vi "BuildMDF.vi"() -> ()   [LabVIEW 2010]
panel:
  out "Draw??":bool
  in  "MDFile":T1
  out "initialized MDF":T2(array[cluster])
  in  "sset/reset MDF":bool
  out "MDF_Original":T2(array[cluster])
  in  "2D Picture":picture
  out "NewMissionDefMap":picture
  in  "Build MDF":bool
  in  "Select Pen Attributes":T3={"Width"=1, "Style"=enum."Solid"}
  in  "Select Your Behavior":T4(ring)
  out "No. of Waypoints":i32
  in  "Path Leg Depth":dbl
  in  "Path Leg Speed":dbl
  out "MissionDefFile":picture
  in  "Pen Color":u32(colorbox)=15671808
  out "Way Point Index":i32
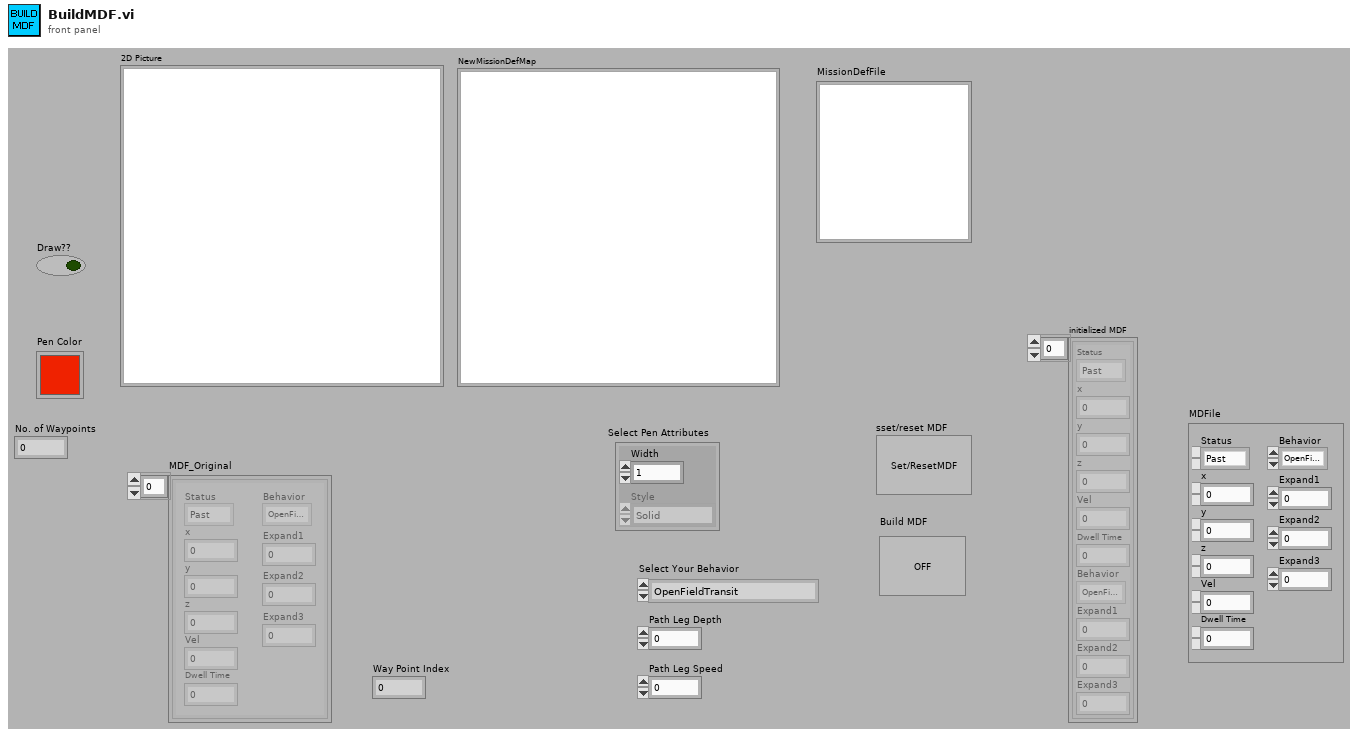
[diagram p1: front panel]
types:
  T1 = cluster{"Status":enum16{"Past", "Current", "Future"}, "x":dbl, "y":dbl, "z":dbl, "Vel":dbl, "Dwell Time":dbl, "Behavior":enum16{"OpenFieldTransit", "WallFollow", "LaneFollow", "ManualMode"}, "Expand1":dbl, "Expand2":dbl, "Expand3":dbl}
  T2 = cluster{"Status":enum16{"Past", "Current", "Future"}, "x":dbl, "y":dbl, "z":dbl, "Vel":dbl, "Dwell Time":dbl, "Behavior":enum16{"OpenFieldTransit", "WallFollow", "LaneFollow", "ManualMode"}, "Expand1":dbl, "Expand2":dbl, "Expand3":dbl}[]
  T3 = cluster{"Width":u16, "Style":enum32{"Solid", "Dash", "Dot", "DashDot", "DashDotDot"}}
  T4 = enum16{"OpenFieldTransit", "WallFollow", "LaneFollow", "ManualMode"}
  T5 = cluster{"Status":enum16{"Past", "Current", "Future"}, "x":dbl, "y":dbl, "z":dbl, "Vel":dbl, "Dwell Time":dbl, "Behavior":enum16{"OpenWaterTransit", "WallFollow", "LaneFollow", "Stop"}, "Expand1":dbl, "Expand2":dbl, "Expand3":dbl}[]
  T6 = enum32{"Solid", "Dash", "Dot", "DashDot", "DashDotDot"}
  T7 = typedef "LVMouseTypeDef.ctl" = cluster{"Mouse Position":cluster{"X":i32, "Y":i32}, "Mouse Modifiers":cluster{"Button Down":bool, "Shift Mod":bool, "Menu Mod":bool, "Option Mod":bool}}
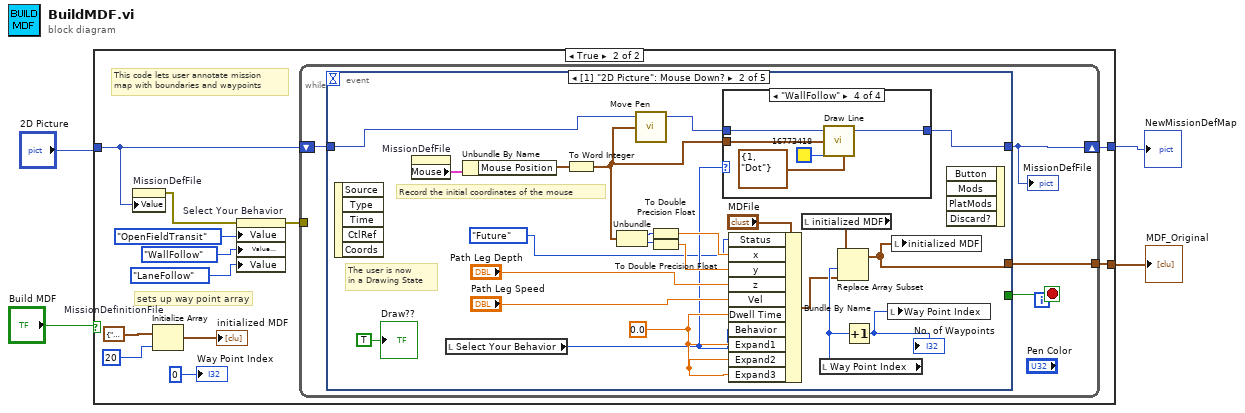
[diagram p0: block diagram]
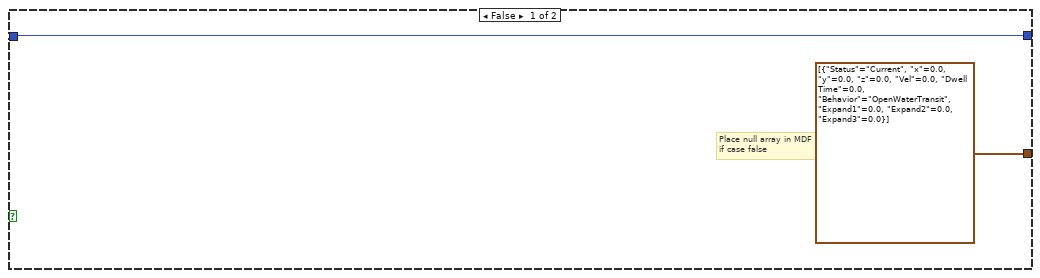
[diagram p2: hidden frame]
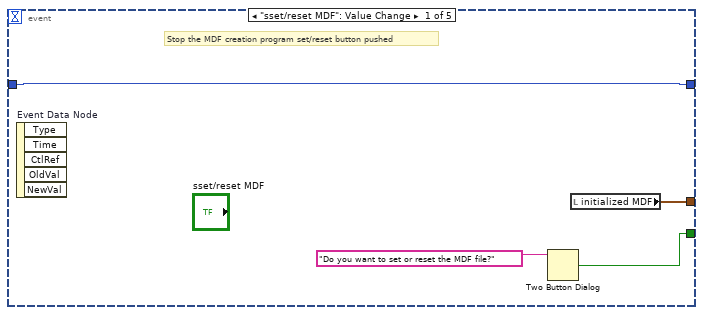
[diagram p3: hidden frame]
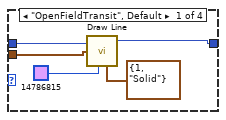
[diagram p4: hidden frame]
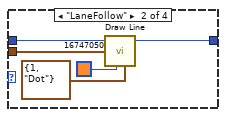
[diagram p5: hidden frame]
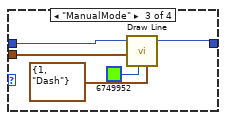
[diagram p6: hidden frame]
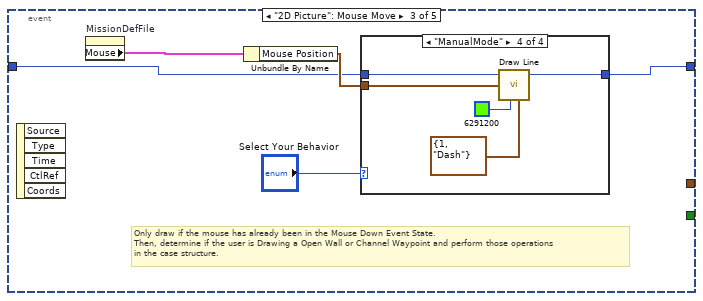
[diagram p7: hidden frame]
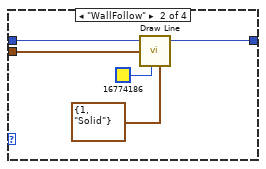
[diagram p9: hidden frame]
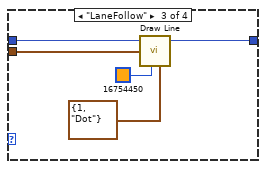
[diagram p10: hidden frame]
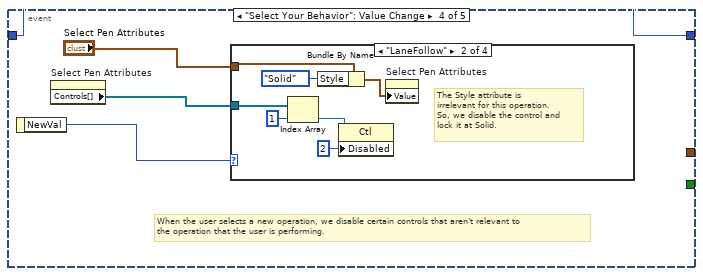
[diagram p11: hidden frame]
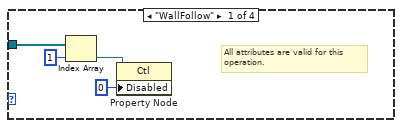
[diagram p12: hidden frame]
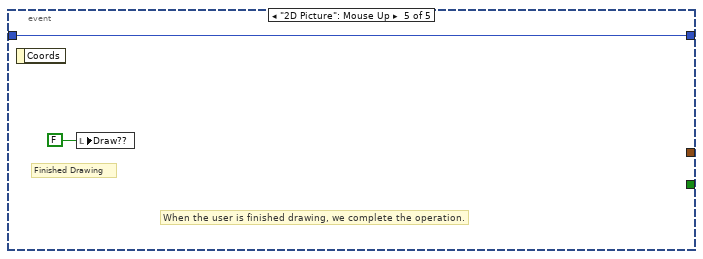
[diagram p15: hidden frame]
diagram:
  n1 = case shown="True" "Build MDF" {
    tunnel: "2D Picture" -> [w6 w16]
    tunnel: [w6 w13] -> w3
    tunnel: [T5 [{"Status"=enum."Current", "x"=0.0, "y"=0.0, "z"=0.0, "Vel"=0.0, "Dwell Time"=0.0, "Behavior"=enum."OpenWaterTransit", "Expand1"=0.0, "Expand2"=0.0, "Expand3"=0.0}] ("MDF_Original") w10] -> w1
    frame False {
      # "Place null array in MDF\nif case false"
    }
    frame True {
      w12 = T1 {"Status"=enum."Current", "x"=0.0, "y"=0.0, "z"=0.0, "Vel"=0.0, "Dwell Time"=0.0, "Behavior"=enum."OpenFieldTransit", "Expand1"=0.0, "Expand2"=0.0, "Expand3"=0.0}  # MissionDefinitionFile
      # "sets up way point array"
      # "This code lets user annotate mission\nmap with boundaries and waypoints"
      n2 = property on="MissionDefFile" class="Pict"("Value"=w16) -> (error out=w17:errorcluster)  [unwired: 2 in, 1 out]
      n3 = Initialize Array ("Initialize WaypointArray")(w12, 20 ("dimension size")) -> (→"initialized MDF":T2)
      n4 = property on="Select Your Behavior" class="Enum (strict)"(error in=w17, "Value"=T4."OpenFieldTransit" ("Select Your Behavior"), "Value (Signaling)"=T4."WallFollow", "Value"=T4."LaneFollow" ("Select Your Behavior")) -> (error out=w18:errorcluster)  [unwired: 1 in, 1 out]
      n5 = while {
        shift-right: [w19] -> w13
        shift-left: w16 -> [w21]
        tunnel: w18 -> [_]
        tunnel: [w20] -> w10
        stop <- w22 stop-if-true
        n6 = event shown="[1] \"2D Picture\": Mouse Down?" {
          selector: _ -> [_ _ _ _ _]
          dyn-events: _ -> [_ _ _ _ _]
          timeout: _ -> [_ _ _ _ _]
          tunnel: [w26 w45 w69 w92 _] -> w19
          tunnel: w21 -> [w26 w43 w70 w92 w106]
          tunnel: [w24 _ _ _ _] -> w22
          tunnel: [w23 w42 _ _ _] -> w20
          tunnel: [_ _ _ _ w106] -> _
          event "sset/reset MDF": Value Change {
            # "Stop the MDF creation program set/reset button pushed"
            n7 = event-data "Event Data Node"() -> ()  [unwired: 1 in, 5 out]
            n8 = Two Button Dialog(message="Do you want to set or reset the MDF file?") -> (T button?=w24:bool)  [unwired: 2 in]
            n9 = local read "initialized MDF"() -> (w23:T2)
          }
          event "2D Picture": Mouse Down? {
            w31 = 0.0 ("Dwell Time")
            # "Record the initial coordinates of the mouse"
            # "The user is now\nin a Drawing State"
            n10 = event-data() -> ()  [unwired: 1 in, 5 out]
            n11 = property on="MissionDefFile" class="Pict"() -> ("Mouse"=w48:T7)  [unwired: 2 in, 2 out]
            n12 = local read "Select Your Behavior"() -> (w30:T4)
            n13 = Unbundle By Name(w48) -> ("Mouse Position"=w44:cluster{"X":i32, "Y":i32})
            n14 = To Word Integer(number=w44) -> (16bit integer=w29:cluster{"X":i16, "Y":i16})
            n15 = Unbundle(w29) -> ("X"=w37:i16, "Y"=w36:i16)
            n16 = call <vilib>:"Move Pen.vi"("new position"=w29, "picture"=w43) -> ("new picture"=w47:picture)  [unwired: 3 in]
            n17 = To Double Precision Float(number=w37) -> (double precision float=w35:dbl)
            n18 = To Double Precision Float(number=w36) -> (double precision float=w34:dbl)
            n19 = case shown="\"WallFollow\"" w30 {
              tunnel: w47 -> [w53 w58 w61 w66]
              tunnel: [w52 w54 w59 w64] -> w45
              tunnel: w29 -> [w51 w57 w60 w65]
              frame "OpenFieldTransit", Default {
                n20 = call <vilib>:"Draw Line.vi"("picture"=w53, "end point"=w51, "color(black)"=u32 14786815, "pen"=T3 {"Width"=1, "Style"=enum."Solid"}) -> ("new picture"=w52:picture)  [unwired: 5 in]
              }
              frame "LaneFollow" {
                n21 = call <vilib>:"Draw Line.vi"("picture"=w58, "end point"=w57, "color(black)"=u32 16747050, "pen"=T3 {"Width"=1, "Style"=enum."Dot"}) -> ("new picture"=w54:picture)  [unwired: 5 in]
              }
              frame "ManualMode" {
                n22 = call <vilib>:"Draw Line.vi"("picture"=w61, "end point"=w60, "color(black)"=u32 6749952, "pen"=T3 {"Width"=1, "Style"=enum."Dash"}) -> ("new picture"=w59:picture)  [unwired: 5 in]
              }
              frame "WallFollow" {
                n23 = call <vilib>:"Draw Line.vi"("picture"=w66, "end point"=w65, "color(black)"=u32 16773418, "pen"=T3 {"Width"=1, "Style"=enum."Dot"}) -> ("new picture"=w64:picture)  [unwired: 5 in]
              }
            }
            n24 = Bundle By Name(cluster="MDFile", "Status"=enum16{"Past", "Current", "Future"}."Future", "x"=w35, "y"=w34, "z"="Path Leg Depth", "Vel"="Path Leg Speed", "Dwell Time"=w31, "Behavior"=w30, "Expand1"=w31, "Expand2"=w31, "Expand3"=w31) -> (w38:T1)
            n25 = local read "initialized MDF"() -> (w40:T2)
            n26 = local read "Way Point Index"() -> (w41:i32)
            n27 = Replace Array Subset(array=w40, new element=w38, index=w41) -> (w42:T2)
            n28 = Increment(x=w41) -> (x+1=w46:i32)
            "No. of Waypoints" <- w46
            n29 = local write "Way Point Index"(w46) -> ()
            n30 = local write "initialized MDF"(w42) -> ()
            n31 = event-data() -> ()  [unwired: 5 in, 1 out]
            "Draw??" <- TRUE ("Draw??")
          }
          event "2D Picture": Mouse Move {
            # "Only draw if the mouse has already been in the Mouse Down Event State.\nThen, determine if the user is Drawing a Open Wall or Channel Waypoint and perform those operations\nin the case structure."
            n32 = event-data() -> ()  [unwired: 1 in, 5 out]
            n33 = property on="MissionDefFile" class="Pict"() -> ("Mouse"=w73:T7)  [unwired: 2 in, 2 out]
            n34 = Unbundle By Name(w73) -> ("Mouse Position"=w71:cluster{"X":i32, "Y":i32})
            n35 = case shown="\"ManualMode\"" "Select Your Behavior" {
              tunnel: w71 -> [_ w78 w83 w86]
              tunnel: [w74 w79 w84 w85] -> w69
              tunnel: w70 -> [w74 w77 w80 w87]
              frame "OpenFieldTransit", Default {
              }
              frame "WallFollow" {
                n36 = call <vilib>:"Draw Line.vi"("picture"=w77, "end point"=w78, "color(black)"=u32 16774186, "pen"=T3 {"Width"=1, "Style"=enum."Solid"}) -> ("new picture"=w79:picture)  [unwired: 5 in]
              }
              frame "LaneFollow" {
                n37 = call <vilib>:"Draw Line.vi"("picture"=w80, "end point"=w83, "color(black)"=u32 16754450, "pen"=T3 {"Width"=1, "Style"=enum."Dot"}) -> ("new picture"=w84:picture)  [unwired: 5 in]
              }
              frame "ManualMode" {
                n38 = call <vilib>:"Draw Line.vi"("picture"=w87, "end point"=w86, "color(black)"=u32 6291200, "pen"=T3 {"Width"=1, "Style"=enum."Dash"}) -> ("new picture"=w85:picture)  [unwired: 5 in]
              }
            }
          }
          event "Select Your Behavior": Value Change {
            # "When the user selects a new operation, we disable certain controls that aren't relevant to\nthe operation that the user is performing."
            n39 = event-data() -> ("NewVal"=w93:T4)  [unwired: 1 in]
            n40 = property on="Select Pen Attributes" class="Clust (strict)"() -> ("Controls[]"=w91:refnum<vi>[])  [unwired: 2 in, 2 out]
            n41 = case shown="\"LaneFollow\"" w93 {
              tunnel: w91 -> [w97 w104 _ _]
              tunnel: "Select Pen Attributes" -> [_ w99 _ _]
              frame "WallFollow" {
                # "All attributes are valid for this\noperation."
                n42 = Index Array "Index Array"(array=w97, index=1) -> (element=w95:refnum<vi>)
                n43 = property on="Property Node" class="Ctl"(reference=w95, "Disabled"=u8 0) -> ()  [unwired: 1 in, 2 out]
              }
              frame "LaneFollow" {
                # "The Style attribute is\nirrelevant for this operation.\nSo, we disable the control and\nlock it at Solid."
                n44 = Index Array(array=w104, index=1) -> (element=w102:refnum<vi>)
                n45 = Bundle By Name(cluster=w99, "Style"=T6."Solid") -> (w98:T3)
                n46 = property class="Ctl"(reference=w102, "Disabled"=u8 2) -> ()  [unwired: 1 in, 2 out]
                n47 = property on="Select Pen Attributes" class="Clust (strict)"("Value"=w98) -> ()  [unwired: 2 in, 2 out]
              }
              frame "OpenFieldTransit" {
              }
              frame "ManualMode" {
              }
            }
          }
          event "2D Picture": Mouse Up {
            # "When the user is finished drawing, we complete the operation."
            # "Finished Drawing"
            n48 = event-data() -> ()  [unwired: 1 in, 1 out]
            n49 = local write "Draw??"(FALSE ("Draw??")) -> ()
          }
        }
        "MissionDefFile" <- w19
      }
      "Way Point Index" <- 0 ("Boundary Point Index")
    }
  }
  "NewMissionDefMap" <- w3
  "MDF_Original" <- w1
